vi "Simple_Inverse_template.vi"(8 "L 2":dbl(slide)=115.0 scale=0.0..200.0, 9 "L 1":dbl(slide)=80.0 scale=0.0..200.0, 11 "end effector":cluster{dbl, dbl}={159.01647214211073, 1.9100783062530127} {"?" format="%.1f"; "?" format="%#.1f"}) -> (0 "Angle 2":dbl(knob)=-72.06882847083946 scale=-90.0..90.0, 1 "Angle1":dbl(knob)=-45.83837436417874 scale=-90.0..90.0)   [LabVIEW 2024]
panel:
  out "2D Picture":picture
  # "mm"
  # "mm"
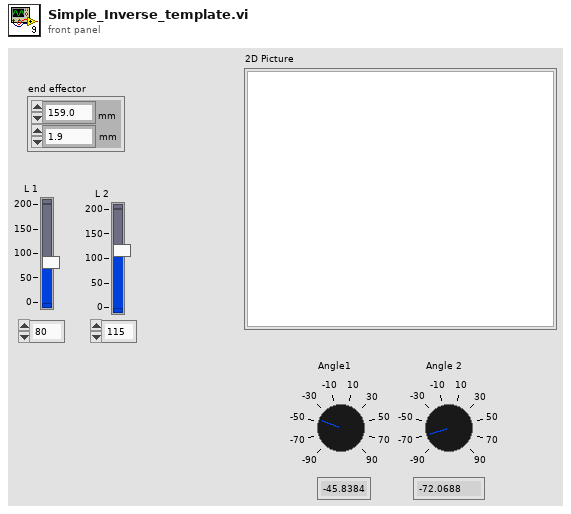
[diagram p1: front panel]
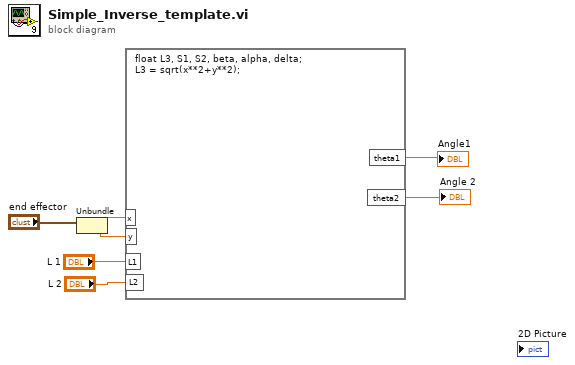
[diagram p0: block diagram]
diagram:
  n1 = Unbundle("end effector") -> (w6:dbl, w5:dbl)
  n2 = formula code="float L3, S1, S2, beta, alpha, delta;\nL3 = sqrt(x**2+y**2);"("L1"="L 1", "L2"="L 2", "x"=w6, "y"=w5) -> ("theta1"=→"Angle1":dbl, "theta2"=→"Angle 2":dbl)
